vi "AlliGator Store Search ROI.vi"(8 "Error In":errorcluster, 11 "Display Image Control Refnum":T2) -> (0 "Error Out":errorcluster, 1 "Message":string, 3 "data":T1)   [LabVIEW 2021, in "AlliGator Source Image.lvlib"]
doc: "Stores Search ROI definition."
uses:
  AlliGator Source Image.lvlib
  Image/Image Control Refnum.ctl
  Globals, Variables, Constants/AlliGator Variables List.ctl
  Image/Image Control ROI Description.ctl
  Variant/Variant to Data/Variant to Boolean.vi
  Globals, Variables, Constants/AlliGator Globals, Variables & Constants.lvlib
  Notebook/AlliGator Notebook.lvlib
  Variant/Variant to Data/Variant to Data.lvlib
  Image/Image.lvlib
  ROIs/AlliGator ROIs.lvlib
panel:
  # "see the AlliGator License on the block diagram (Ctrl+E or Window:Show Block Diagram)"
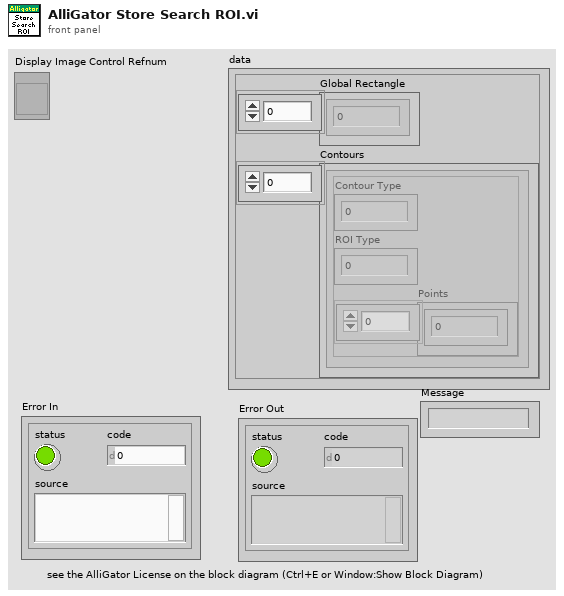
[diagram p1: front panel]
types:
  T1 = cluster{"Global Rectangle":i32[], "Contours":cluster{"Contour Type":u32, "ROI Type":u32, "Points":i32[]}[]}
  T2 = typedef "Image.lvlib/Image Control Refnum.ctl" = refnum<vi>
  T3 = typedef "AlliGator Globals, Variables & Constants.lvlib/AlliGator Variables List.ctl" = enum16{"---- GUI ----", "GUI:Initialization Status", "GUI:State Indicators Refnum", "GUI:Original AlliGator Menu Items", "GUI:Current Action Loop State", "GUI:Script in progress", "GUI:Playback", "GUI:Loop Playback", "GUI:Search ROI Used", "GUI:Search ROI", "Decay Graph Max Legend Size", "Intensity Graph Max Legend Size", "Decay Statistics Graph Max Legend Size", "Phasor Graph Max Legend Size", "Phasor Ratio Graph Max Legend Size", "Lifetime Graph Max Legend Size", "---- Files ----", "Files:Export Dataset Frames as Individual Files", "Files:Show Batch Export Help Balloons", "Files:Frames in Dataset", "Files:ptu File Frame Start Indices", "Files:Current Frame in Dataset", "Files:Current Frame Timestamp", "Files:Dataset Loaded", "Files:Dataset Metadata", "Files:Dataset Channel", "Files:Dataset Data Description", "Files:Background Dataset Metadata", "Files:Background Dataset Channel", "Files:Background Dataset Data Description", "Files:Background File Subtraction", "Files:Background File Path", "Files:Background File Pile-up Correction", "Files:Background File Pixel Well Capacity", "Files:Background File Scaling Factor", "Files:Current Dataset Load Settings", "Files:Dataset Path", "Files:ICCD-specific Information", "Files:Macrotime Gate Separation", "------ Python Plugins ------", "Python Plugins:Information", "Python Plugins:Python Session", "Python Plugins:Valid Python Session?", "---- Source Image ----", "Source Image:ROIs", "Source Image:Current ROI", "Source Image:ROI Event Refnum", "X_Source Image Display Range", "X_Source Image Palette Information", "X_Type of Displayed Image", "X_Time Gate Slider", "Source Image:Palette List", "Source Image:Scale", "Source Image:ROI Overlay Color", "Source Image:Overlay to Erase", "Source Image:Is Displayed Image Accumulated", "Source Image:White Light Image Modified", "Source Image:Mask Image Modified", "---- Image Profile Window ----", "Image Profile:Window Event Refnum", "Image Profile:IntensityType", "Image Profile:Intensity Average Type", "Image Profile:Intensity-weighted SDV", "Image Profile:Box Profile Type", "Image Profile:Window Open", "Image Profile:Plotted Fit Parameter", "------ Phasor Graph -------", "Phasor Graph:Show Line", "---- Phasor Plot ---", "Phasor Plot:Parameters Changed", "Phasor Plot:FLI Dataset Modified since last Calculation", "Phasor Harmonics Data", "Selected Phasor Harmonics", "Phasor Harmonic Manager Event Refnum", "Phasor Plot:ROIs", "Phasor Plot:Current ROI", "Phasor Plot:ROI Event Refnum", "Phasor Plot:Image Reference Points", "Phasor Plot:Computed", "Phasor Plot:Palette Information", "Phasor Plot:Palette List", "Phasor Plot:Phasor Ratio Palette Information", "Phasor Plot:Phasor Ratio Palette List", "Phasor Plot:Image Scale", "Phasor Plot:Image Overlay to Erase", "Phasor Plot:Image Elements to Update", "Phasor Plot:Current Calculation Parameters", "Phasor Plot:Current Calibration Options", "Phasor Plot:Reset Cumulated Phasor Plot", "Phasor Plot:Reference 1", "Phasor Plot:Lifetime Reference 1", "Phasor Plot:Reference 1 Frequency", "Phasor Plot:Reference 2", "Phasor Plot:Lifetime Reference 2", "Phasor Plot:Reference 2 Frequency", "---- Decay Analysis ----", "Number of Selected Decays to Fit", "LS Fit Results", "LAR Fit Results", "BS Fit Results", "Last Decay Max - Min", "Best Fit Parameters", "Best Fit Parameter Names", "Actual Size X", "Actual Size Y", "Binning X", "Binning Y", "Actual # Gates", "Dataset Number", "Gates to...", "Gates Skipped", "Gates to keep", "Gate Step", "Gate Separation", "Reversed Gates", "Pile-up Correction", "Pixel Well Capacity", "Background Subtracted", "Background Subtraction Method", "Background Definition Range", "Background File (deprecated)", "Number of Dataset Accumulated", "Array of Accumulated Dataset Paths", "Do Averaged Datasets", "Destination File Path", "Process Plot Target", "Use 1/D as Phasor Frequency", "---- Decay Fit Parameter Map -----", "Decay Fit Parameter Map:Palette Information", "Decay Fit Parameter Map:Palette List", "---- Parameter Map ----", "Parameter Map:Palette Information", "Parameter Map:Palette List", "------- Local Decay Window ---------", "Local Decay Graph Window:Event Refnum", "Local Decay Graph Window:Use normalized IRF for convolution", "----- Miscellaneous ----", "Misc:Skippable Dialog Windows Status"}
  T4 = typedef "Image.lvlib/Image Control ROI Description.ctl" = cluster{"Image Control Label":string, "ROI Descriptor":T5}
  T5 = typedef "ROI Descriptor" = cluster{"Global Rectangle":i32[], "Contours":cluster{"ID":enum32{"External", "Internal"}, "Type":u32, "Coordinates":i32[]}[]}
  T6 = typedef "Image.lvlib/Image Control ROI Description v2.ctl" = cluster{"Image Control Label":string, "Named ROI Description":T7}
  T7 = typedef "Image.lvlib/Named ROI Description.ctl" = cluster{"ROI Descriptor":T5, "ROI Name":string, "Overlay Color":u32}
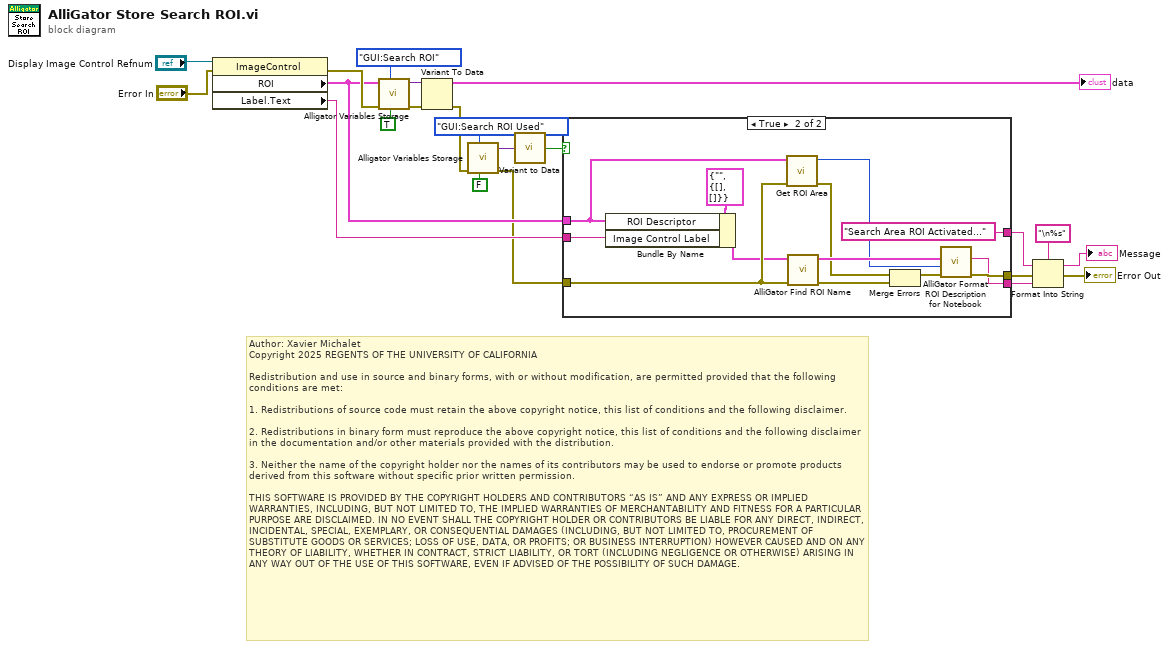
[diagram p0: block diagram]
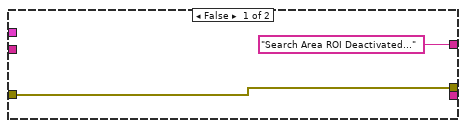
[diagram p2: hidden frame]
diagram:
  # "Author: Xavier Michalet\nCopyright 2025 REGENTS OF THE UNIVERSITY OF CALIFORNIA\n\nRedistribution and use in source and binary forms, with or without modification, are permitted provided that the following conditions are met:\n\n1. Redistributions of source code must retain the above copyright notice, this list of conditions and the following disclaimer.\n\n2. Redistributions in binary form must reproduce the above copyright notice, this list of conditions and the following disclaimer in the documentation and/or other materials provided with the distribution.\n\n3. Neither the name of the copyright holder nor the names of its contributors may be used to endorse or promote products derived from this software without specific prior written permission.\n\nTHIS SOFTWARE IS PROVIDED BY THE COPYRIGHT HOLDERS AND CONTRIBUTORS “AS IS” AND ANY EXPRESS OR IMPLIED WARRANTIES, INCLUDING, BUT NOT LIMITED TO, THE IMPLIED WARRANTIES OF MERCHANTABILITY AND FITNESS FOR A PARTICULAR PURPOSE ARE DISCLAIMED. IN NO EVENT SHALL THE COPYRIGHT HOLDER OR CONTRIBUTORS BE LIABLE FOR ANY DIRECT, INDIRECT, INCIDENTAL, SPECIAL, EXEMPLARY, OR CONSEQUENTIAL DAMAGES (INCLUDING, BUT NOT LIMITED TO, PROCUREMENT OF SUBSTITUTE GOODS OR SERVICES; LOSS OF USE, DATA, OR PROFITS; OR BUSINESS INTERRUPTION) HOWEVER CAUSED AND ON ANY THEORY OF LIABILITY, WHETHER IN CONTRACT, STRICT LIABILITY, OR TORT (INCLUDING NEGLIGENCE OR OTHERWISE) ARISING IN ANY WAY OUT OF THE USE OF THIS SOFTWARE, EVEN IF ADVISED OF THE POSSIBILITY OF SUCH DAMAGE."
  n1 = property class="ImageControl"(reference="Display Image Control Refnum", error in="Error In") -> (error out=w21:errorcluster, "ROI"=w16:T1, "Label.Text"=w15:string)  [unwired: 1 out]
  n2 = call "Alligator Variables Storage.vi"("Get(F)/Set"=TRUE, "AlliGator Variable"=AlliGator_Variables_List."GUI:Search ROI" ("Alligator Variable"), "Error In"=w21, "Data in"=w16) -> ("Error Out"=w14:errorcluster, "Data out"=w18:variant)  [unwired: 5 in, 1 out]
  n3 = Variant To Data(error in=w14, Variant=w18) -> (data=→"data":T1, error out=w7:errorcluster)  [unwired: 1 in]
  n4 = call "Alligator Variables Storage.vi"("Get(F)/Set"=FALSE, "AlliGator Variable"=AlliGator_Variables_List."GUI:Search ROI Used" ("Alligator Variable"), "Error In"=w7) -> ("Error Out"=w11:errorcluster, "Data out"=w10:variant)  [unwired: 6 in, 1 out]
  n5 = call-poly "Variant to Data.vi"("Variant"=w10) -> ("Value"=w9:bool)  [unwired: 8 in]
  n6 = case shown="True" w9 {
    tunnel: w16 -> [_ w32]
    tunnel: w15 -> [_ w36]
    tunnel: w11 -> [w24 w35]
    tunnel: [w24 w27] -> w6
    tunnel: ["Search Area ROI Deactivated..." ("Message") "Search Area ROI Activated..." ("Message")] -> w4
    tunnel: [_ w25] -> w2
    frame False {
    }
    frame True {
      n7 = Bundle By Name(cluster=T4 {"Image Control Label"="", "ROI Descriptor"={"Global Rectangle"=[], "Contours"=[]}} ("Image Control ROI Description"), "ROI Descriptor"=w32, "Image Control Label"=w36) -> (w30:T4)
      n8 = call "Get ROI Area.vi"("Error In"=w35, "ROI Descriptor"=w32) -> ("Error Out"=w28:errorcluster, "Number of Pixels"=w31:u32)  [unwired: 8 in]
      n9 = call "AlliGator Find ROI Name.vi"("Error In"=w35, "ROI Descriptor"=w30) -> ("Error Out"=w34:errorcluster, "Image Control ROI Description"=w33:T6)  [unwired: 7 in, 1 out]
      n10 = Merge Errors(w28, w34) -> (w29:errorcluster)
      n11 = call "AlliGator Format ROI Description for Notebook.vi"("error in (no error)"=w29, "# Pixels"=w31, "ROI Descriptor"=w33) -> ("error out"=w27:errorcluster, "Message"=w25:string)  [unwired: 7 in]
    }
  }
  n12 = Format Into String(format string="\n%s", initial string=w4, error in=w6, w2) -> (resulting string=→"Message":string, error out=→"Error Out":errorcluster)
